vi "Channel Measurement Fetch Complex.vi"(0 "instrument handle":refnum<k15>, 5 "RepCapIdentifier":string, 9 "ValBufferSize":i32=2048, 11 "error in (no error)":errorcluster {"code" format="%.0x"}) -> (4 "instrument handle out":refnum<k15>, 6 "Val":dbl[](array[numeric]) format="%.2p", 8 "ValActualSize":i32, 15 "error out":errorcluster {"code" format="%.0x"})   [LabVIEW 2014, in "Agilent NA.lvlib"]
doc: "Returns real and imaginary values of measurement data"
uses:
  Agilent NA.lvlib
  AgNA.dll
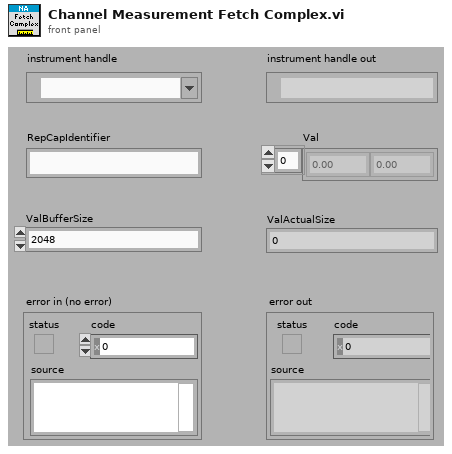
[diagram p1: front panel]
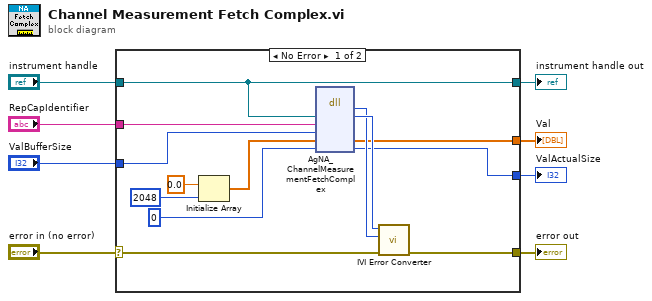
[diagram p0: block diagram]
diagram:
  n1 = case shown="No Error" "error in (no error)" {
    selector: "error in (no error)" -> [w19 w23]
    tunnel: [w18 w23] -> w8
    tunnel: "RepCapIdentifier" -> [w17 _]
    tunnel: [w14 _] -> w5
    tunnel: [w12 _] -> w4
    tunnel: [w11 w22] -> w3
    tunnel: "instrument handle" -> [w11 w22]
    tunnel: "ValBufferSize" -> [w10 _]
    frame No Error {
      n2 = Initialize Array(0.0 ("element"), 2048 ("pRealResponseValActualSize")) -> (w16:dbl[])
      n3 = dll-call lib="AgNA**.dll" fn="AgNA_ChannelMeasurementFetchComplex"("Vi"=w11, "RepCapIdentifier"=w17, "ValBufferSize"=w10, "Val"=w16, "ValActualSize"=0 ("pRealResponseValActualSize")) -> ("return type"=w20:i32, "Vi"=w21:u32, "Val"=w14:sgl[], "ValActualSize"=w12:i32)  [unwired: 5 in, 2 out]
      n4 = call "IVI Error Converter.vi"("error in (no error)"=w19, "IVI error code (0)"=w20, "instrument handle"=w21) -> ("error out"=w18:errorcluster)  [unwired: 7 in, 1 out]
    }
    frame Error {
    }
  }
  "error out" <- w8
  "instrument handle out" <- w3
  "Val" <- w5
  "ValActualSize" <- w4
